vi "Wrap Position To World.vi"(11 "Position":refnum<class "Vector 2D.lvclass">) -> (3 "Position Wrapped To World":refnum<class "Vector 2D.lvclass">)   [LabVIEW 2021]
uses:
  Re-use Libraries/Vector 2D/Vector 2D.lvclass
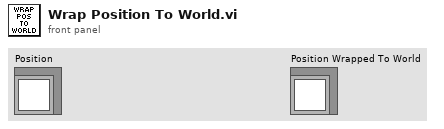
[diagram p1: front panel]
types:
  T1 = typedef "Constants.ctl" = cluster{"Colours":cluster{"OK":u32, "Warning":u32, "Error":u32, "Red":u32, "Green":u32, "Blue":u32, "Yellow":u32}, "System":cluster{"Target Frames Second":dbl, "World Size":T2, "Window Size":T2, "Battle Area Size":T2, "Sidebar Scaling":sgl, "Sidebar Width":i32, "SC2 Frame Rate [Seconds/Frame]":sgl}, "Game":cluster{"Maximum Asteroids":i32, "Max Energy":i32, "Max Crew":i32, "Maximum Stars":i32}}
  T2 = typedef "SDL2 Utility.lvlib/Point (I32).ctl" = cluster{"x":i32, "y":i32}
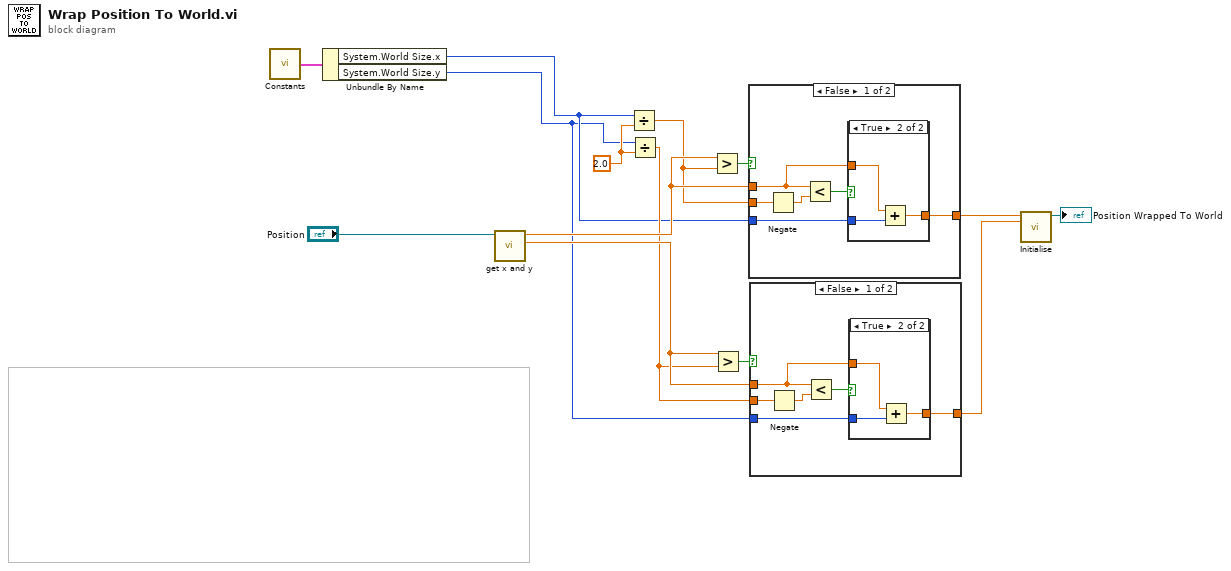
[diagram p0: block diagram]
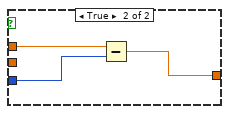
[diagram p3: hidden frame]
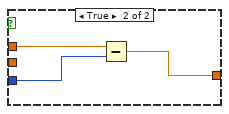
[diagram p5: hidden frame]
diagram:
  w13 = sgl 2.0 ("y")
  n1 = call "Constants.vi"() -> ("Constants"=w4:T1)
  n2 = Unbundle By Name(w4) -> ("System.World Size.x"=w3:i32, "System.World Size.y"=w2:i32)
  n3 = call "get x and y.vi"("Vector 2D in"="Position") -> ("y"=w8:sgl, "x"=w11:sgl)  [unwired: 9 in]
  n4 = Divide(x=w3, y=w13) -> (x/y=w6:sgl)
  n5 = Divide(x=w2, y=w13) -> (x/y=w5:sgl)
  n6 = Greater?(x=w11, y=w6) -> (0:w12:bool)
  n7 = Greater?(x=w8, y=w5) -> (0:w9:bool)
  n8 = case shown="False" w12 {
    tunnel: w11 -> [w18 w27]
    tunnel: w3 -> [w16 w26]
    tunnel: [w17 w25] -> w10
    tunnel: w6 -> [w15 _]
    frame False {
      n9 = Negate(x=w15) -> (-x=w20:sgl)
      n10 = Less?(x=w18, y=w20) -> (x < y?=w19:bool)
      n11 = case shown="True" w19 {
        tunnel: w18 -> [w21 w24]
        tunnel: [w21 w23] -> w17
        tunnel: w16 -> [_ w22]
        frame False {
        }
        frame True {
          n12 = Add(x=w24, y=w22) -> (x+y=w23:sgl)
        }
      }
    }
    frame True {
      n13 = Subtract(x=w27, y=w26) -> (x-y=w25:sgl)
    }
  }
  n14 = case shown="False" w9 {
    tunnel: w8 -> [w31 w40]
    tunnel: w2 -> [w29 w39]
    tunnel: [w30 w38] -> w7
    tunnel: w5 -> [w28 _]
    frame False {
      n15 = Negate(x=w28) -> (-x=w33:sgl)
      n16 = Less?(x=w31, y=w33) -> (x < y?=w32:bool)
      n17 = case shown="True" w32 {
        tunnel: w31 -> [w34 w37]
        tunnel: [w34 w36] -> w30
        tunnel: w29 -> [_ w35]
        frame False {
        }
        frame True {
          n18 = Add(x=w37, y=w35) -> (x+y=w36:sgl)
        }
      }
    }
    frame True {
      n19 = Subtract(x=w40, y=w39) -> (x-y=w38:sgl)
    }
  }
  n20 = call "Initialise.vi"("y"=w7, "x"=w10) -> ("Vector 2D out"=→"Position Wrapped To World":refnum<class "Vector 2D.lvclass">)  [unwired: 9 in]
